vi "Datalog to ASCII (DATA, Mode 0).vi"(4 "Error in":errorcluster, 5 "ASCII output path":path=path "C:/Datalogs/Log1_P0.txt", 6 "Precision":i16=4, 7 "Datalog path":path=path "C:/Datalogs/Log1_P0.log") -> (0 "Error out":errorcluster)   [LabVIEW 2015]
uses:
  Ctls/Data values, Mode 0 (for datalog).ctl
  <vilib>/Utility/file.llb/Write Delimited Spreadsheet (string).vi
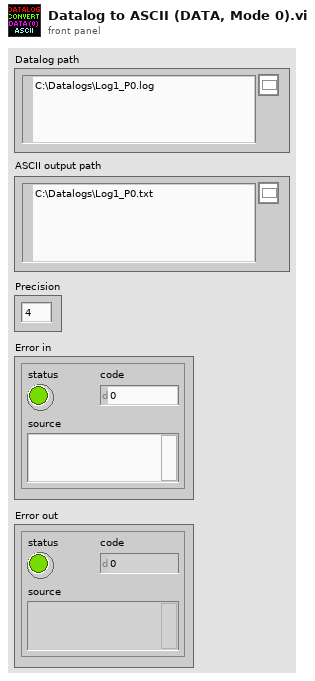
[diagram p1: front panel]
types:
  T1 = typedef "Data values, Mode 0 (for datalog).ctl" = cluster{"Time Stamp":timestamp, "dt (us)":sgl, "dt_warn":u8, "Pressures":sgl[], "Statuses":u8[]}
  T2 = enum16{"open", "replace", "create", "open or create", "replace or create", "replace or create with confirmation"}
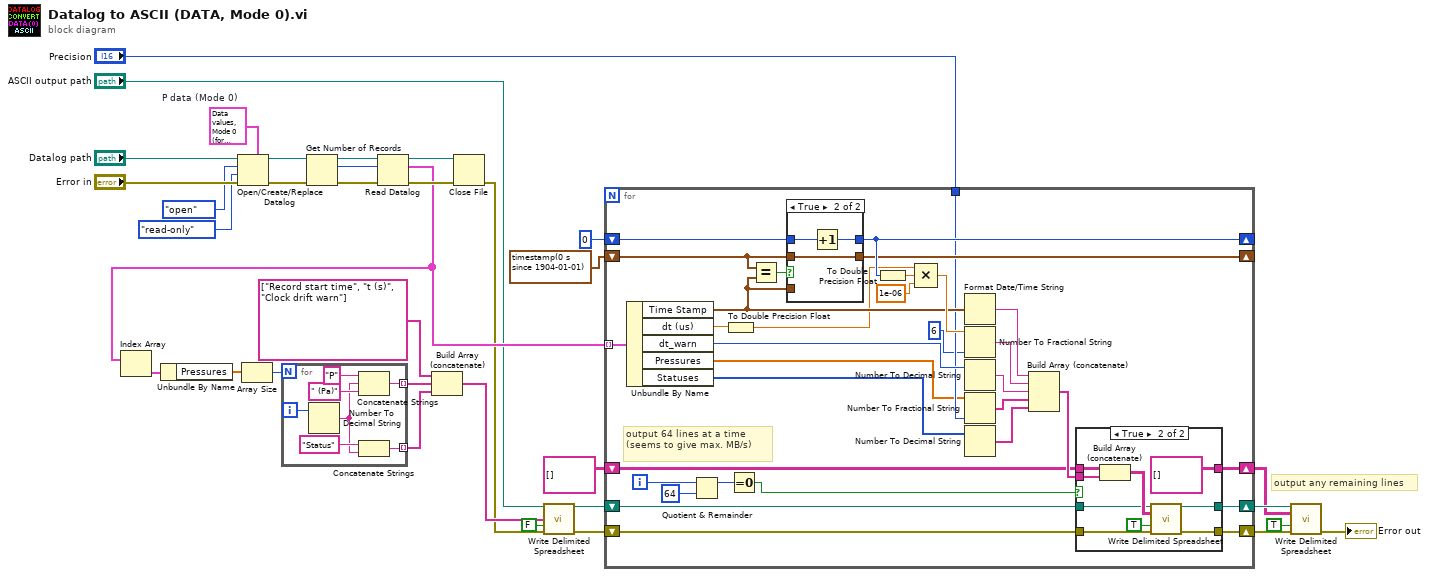
[diagram p0: block diagram]
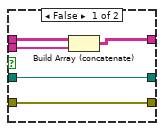
[diagram p2: hidden frame]
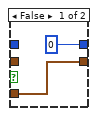
[diagram p3: hidden frame]
diagram:
  w21 = T1 {"Time Stamp"=timestamp(0 s since 1904-01-01), "dt (us)"=0.0, "dt_warn"=0, "Pressures"=[], "Statuses"=[]}  # P data (Mode 0)
  # "output any remaining lines"
  n1 = Open/Create/Replace Datalog(5:w21, 8:"Error in", 9:enum16{"read/write", "read-only", "write-only"}."read-only" ("access (0:read/write)"), 10:T2."open" ("operation (0:open)"), 11:"Datalog path") -> (0:w29:errorcluster, 3:w30:refnum<k1>)  [unwired: 1 in, 1 out]
  n2 = Get Number of Records(4:w29, 7:w30) -> (0:w26:errorcluster, 2:w27:i64, 3:w28:refnum<k1>)
  n3 = Read Datalog(4:w26, 6:w27, 7:w28) -> (0:w24:errorcluster, 2:w16:T1[], 3:w25:refnum<k1>)
  n4 = Index Array(array=w16) -> (element=w15:T1)  [unwired: 1 in]
  n5 = Unbundle By Name(w15) -> ("Pressures"=w14:sgl[])
  n6 = Array Size(array=w14) -> (size(s)=w13:i32)
  n7 = for {
    N: w13 -> [_]
    tunnel: [w36] -> w19 mode=indexing
    tunnel: [w35] -> w18 mode=indexing
    i -> [w41]
    n8 = Number To Decimal String(number=w41) -> (decimal integer string=w37:string)  [unwired: 1 in]
    n9 = Concatenate Strings("P", w37, " (Pa)") -> (w36:string)
    n10 = Concatenate Strings("Status", w37) -> (w35:string)
  }
  n11 = Build Array (concatenate)(string[] ["Record start time", "t (s)", "Clock drift warn"], w19, w18) -> (w3:string[])
  n12 = Close File(refnum=w25, error in=w24) -> (error out=w2:errorcluster)  [unwired: 1 out]
  n13 = call-poly <vilib>:"Write Delimited Spreadsheet.vi"("file path (dialog if empty)"="ASCII output path", "1D data"=w3, "append to file? (F)"=FALSE, "error in (no error)"=w2) -> ("new file path (Not A Path if cancelled)"=w10:path, "error out"=w9:errorcluster)  [unwired: 10 in]
  n14 = for {
    tunnel: w16 -> [w64] mode=indexing
    shift-right: [w66] -> _
    shift-left: u32 0 -> [w67]
    shift-right: [w65] -> _
    shift-left: timestamp(0 s since 1904-01-01) ("Time stamp") -> [w68]
    tunnel: "Precision" -> [w58]
    shift-right: [w44] -> w7
    shift-left: w9 -> [w45]
    shift-right: [w43] -> w8
    shift-left: w10 -> [w46]
    shift-right: [w48] -> w6
    shift-left: string[][] [] -> [w49]
    i -> [w51]
    # "output 64 lines at a time (seems to give max. MB/s)"
    n15 = Unbundle By Name(w64) -> ("Time Stamp"=w63:timestamp, "dt (us)"=w62:sgl, "dt_warn"=w60:u8, "Pressures"=w57:sgl[], "Statuses"=w54:u8[])
    n16 = Quotient & Remainder(x=w51, y=64) -> (x-y*floor(x/y)=w53:i32)  [unwired: 1 out]
    n17 = To Double Precision Float(number=w62) -> (double precision float=w61:dbl)
    n18 = Equal To 0?(x=w53) -> (x = 0?=w47:bool)
    n19 = Equal?(x=w68, y=w63) -> (x = y?=w69:bool)
    n20 = case shown="True" w69 {
      tunnel: [u32 0 w92] -> w66
      tunnel: w67 -> [_ w91]
      tunnel: w63 -> [w90 _]
      tunnel: w68 -> [_ w93]
      tunnel: [w90 w93] -> w65
      frame False {
      }
      frame True {
        n21 = Increment(x=w91) -> (x+1=w92:u32)
      }
    }
    n22 = To Double Precision Float(number=w66) -> (double precision float=w74:dbl)
    n23 = Compound Arithmetic op=MULTIPLY(w61, w74, 1e-06 ("value")) -> (w72:dbl)
    n24 = Format Date/Time String(seconds (now)=w63) -> (date/time string=w73:string)  [unwired: 2 in]
    n25 = Number To Fractional String(number=w72, precision (6)=i16 6) -> (F-format string=w71:string)  [unwired: 2 in]
    n26 = Number To Decimal String(number=w60) -> (decimal integer string=w59:string)  [unwired: 1 in]
    n27 = Number To Fractional String(number=w57, precision (6)=w58) -> (F-format string=w56:string[])  [unwired: 2 in]
    n28 = Number To Decimal String(number=w54) -> (decimal integer string=w55:string[])  [unwired: 1 in]
    n29 = Build Array (concatenate)(w73, w71, w59, w56, w55) -> (w50:string[])
    n30 = case shown="True" w47 {
      tunnel: [w79 string[][] []] -> w48
      tunnel: [w76 w87] -> w43
      tunnel: [w75 w86] -> w44
      tunnel: w50 -> [w77 w83]
      tunnel: w49 -> [w78 w82]
      tunnel: w46 -> [w76 w81]
      tunnel: w45 -> [w75 w80]
      frame False {
        n31 = Build Array (concatenate)(w78, w77) -> (w79:string[][])
      }
      frame True {
        n32 = Build Array (concatenate)(w82, w83) -> (w84:string[][])
        n33 = call-poly <vilib>:"Write Delimited Spreadsheet.vi"("file path (dialog if empty)"=w81, "2D data"=w84, "append to file? (F)"=TRUE, "error in (no error)"=w80) -> ("new file path (Not A Path if cancelled)"=w87:path, "error out"=w86:errorcluster)  [unwired: 10 in]
      }
    }
  }
  n34 = call-poly <vilib>:"Write Delimited Spreadsheet.vi"("file path (dialog if empty)"=w8, "2D data"=w6, "append to file? (F)"=TRUE, "error in (no error)"=w7) -> ("error out"=→"Error out":errorcluster)  [unwired: 10 in, 1 out]
